vi "Assign Point Values to Grid.vi"(8 "error in (no error)":errorcluster, 10 "Point Value of Difficulty Levels":i32[](array[numeric]), 11 "Grid Screen in":refnum<class "Grid Screen.lvclass">) -> (0 "error out":errorcluster, 3 "Grid Screen out":refnum<class "Grid Screen.lvclass">)   [LabVIEW 2021, in "Grid Screen.lvlib" / "Grid Screen.lvclass"]
uses:
  Grid Screen.lvclass
  Grid Screen.lvclass/Grid Screen.ctl
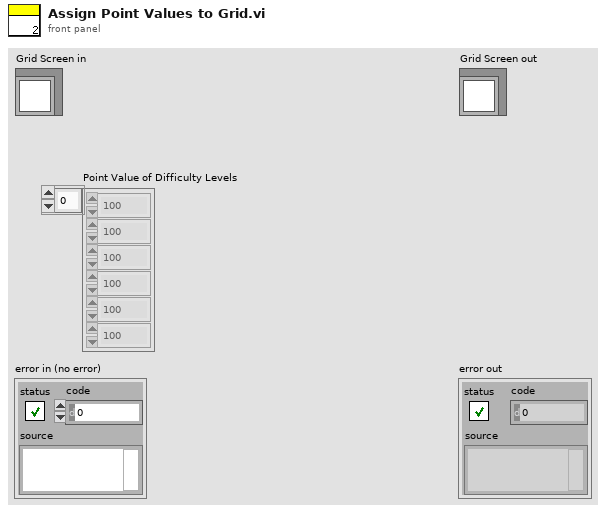
[diagram p1: front panel]
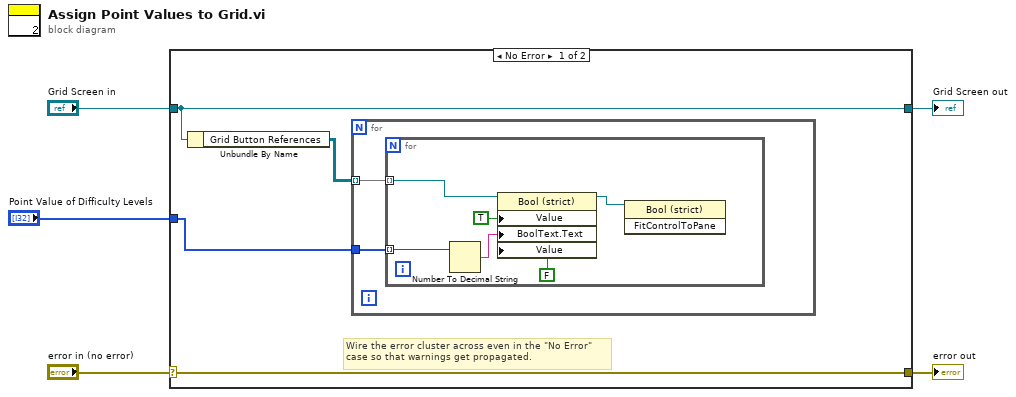
[diagram p0: block diagram]
diagram:
  n1 = case shown="No Error" "error in (no error)" {
    selector: "error in (no error)" -> [w9 w19]
    tunnel: [w9 w19] -> w4
    tunnel: [w8 w18] -> w2
    tunnel: "Grid Screen in" -> [w8 w18]
    tunnel: "Point Value of Difficulty Levels" -> [w6 _]
    frame No Error {
      # "Wire the error cluster across even in the \"No Error\"\ncase so that warnings get propagated."
      n2 = Unbundle By Name(w8) -> ("Grid Button References"=w7:refnum<vi>[][])
      n3 = for {
        tunnel: w7 -> [w11] mode=indexing
        tunnel: w6 -> [w10]
        n4 = for {
          tunnel: w11 -> [w17] mode=indexing
          tunnel: w10 -> [w16] mode=indexing
          n5 = Number To Decimal String(number=w16) -> (decimal integer string=w14:string)  [unwired: 1 in]
          n6 = property class="Bool (strict)"(reference=w17, "Value"=TRUE, "BoolText.Text"=w14, "Value"=FALSE) -> (reference out=w15:refnum<vi>)  [unwired: 1 in, 1 out]
          n7 = invoke class="Bool (strict)" method="FitControlToPane"(reference=w15) -> ()  [unwired: 2 in, 3 out]
        }
      }
    }
    frame Error {
    }
  }
  "error out" <- w4
  "Grid Screen out" <- w2
